vi "Roll station.vi"(0 "configuration file path":path caption="配置文件的路径", 1 "Roll station msic inf":T1) -> ()   [LabVIEW 2014]
uses:
  Ctl.xio/Roll station msic ctl.ctl
  SubVIS.xio/DataSocket/DataSocket_Tags.ctl
  Ctl.xio/part type.ctl
  SubVIS.xio/Creat Write List VI's/DefCtrl/Station.ctl
  <vilib>/Utility/file.llb/Read From Spreadsheet File (string).vi
  SubVIS.xio/Hopper car inf/Curing inf.vi
  SubVIS.xio/DataSocket/Write PLC Vars/Write Dbl Var in.vi
  SubVIS.xio/DataSocket/Write PLC Vars/Write Bool Var in.vi
panel:
  in  "SQL information":string
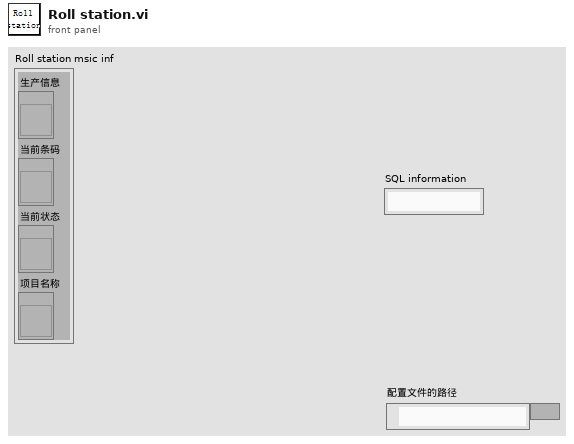
[diagram p1: front panel]
types:
  T1 = cluster{"生产信息":refnum<vi>, "当前条码":refnum<vi>, "当前状态":refnum<vi>, "项目名称":refnum<vi>}
  T2 = typedef "Station.ctl" = enum16{"粗切工位", "热处理工位", "精切工位", "PDF焊接工位", "打凹点预载力工位", "收卷工位", "EOL工位"}
  T3 = typedef "Roll station msic ctl.ctl" = cluster{"configuration file path":path, "DsOut":T4[], "Hopper car information":cluster{"Hopper car code":string, "Hopper car No":string, "plate No":string}, "pallet.produced number":i32, "SQL information":string, "Serial number":i32, "database path":path, "Roll station msic inf":cluster{"生产信息":refnum<vi>, "当前条码":refnum<vi>, "当前状态":refnum<vi>, "项目名称":refnum<vi>}, "part type":T5, "BarCode":string, "scanner resource name out":refnum<visa-resource-name>, "scanner coms or ip":string, "scanner ip ID":refnum<k5>, "curing timer":i32}
  T4 = typedef "DataSocket_Tags.ctl" = cluster{"Ds ID":refnum<k13>, "Tag":string}
  T5 = typedef "part type.ctl" = cluster{"项目号":string, "物料代码":string, "零件号":string, "供应商编码":string, "产线编码":string, "客户代码":string, "颜色代码":string, "托盘上限":i32, "加热温度":string, "加热时长":string, "EOL Stations":string}
  T6 = cluster{"Hopper car code":string, "Hopper car No":string, "plate No":string}
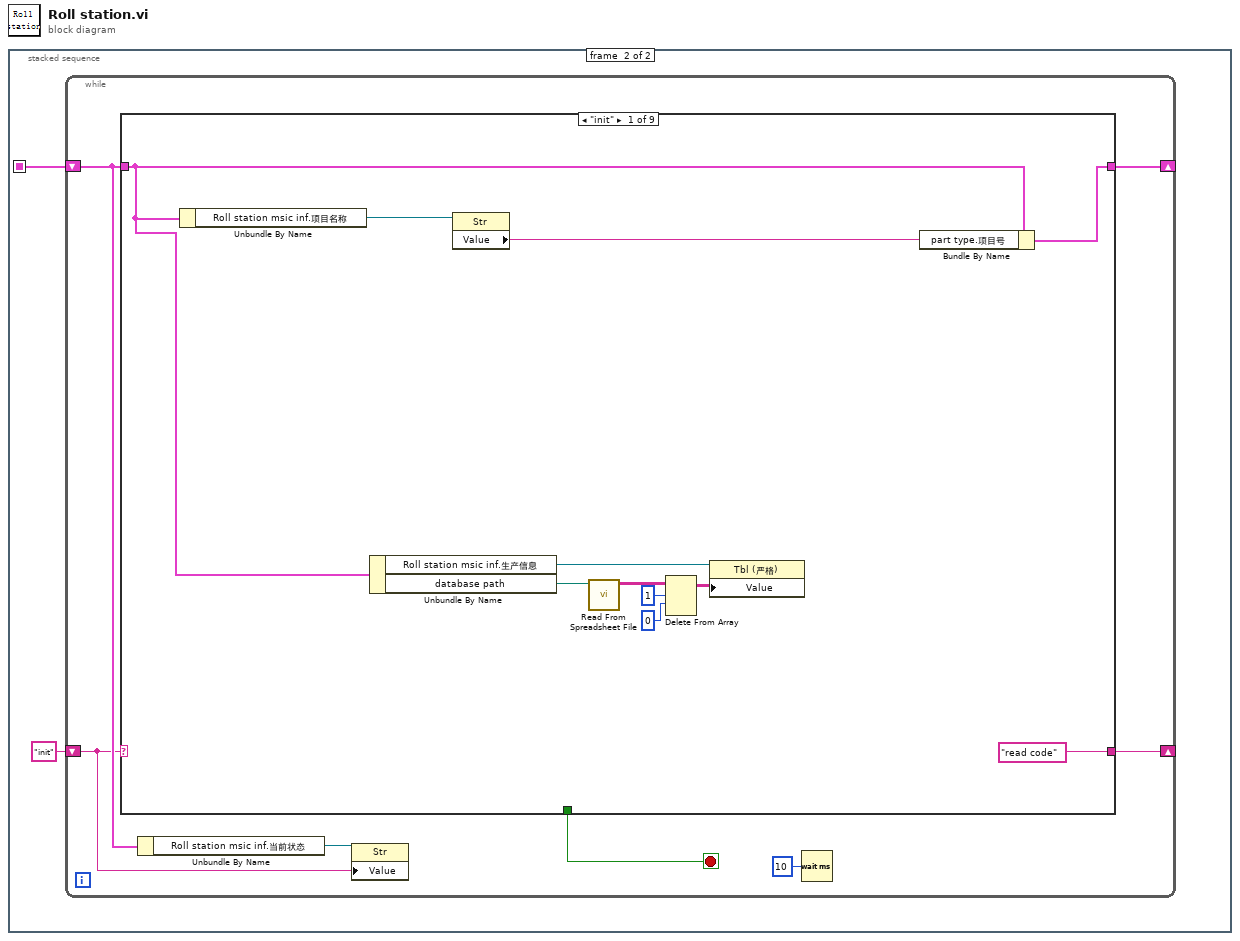
[diagram p0: block diagram]
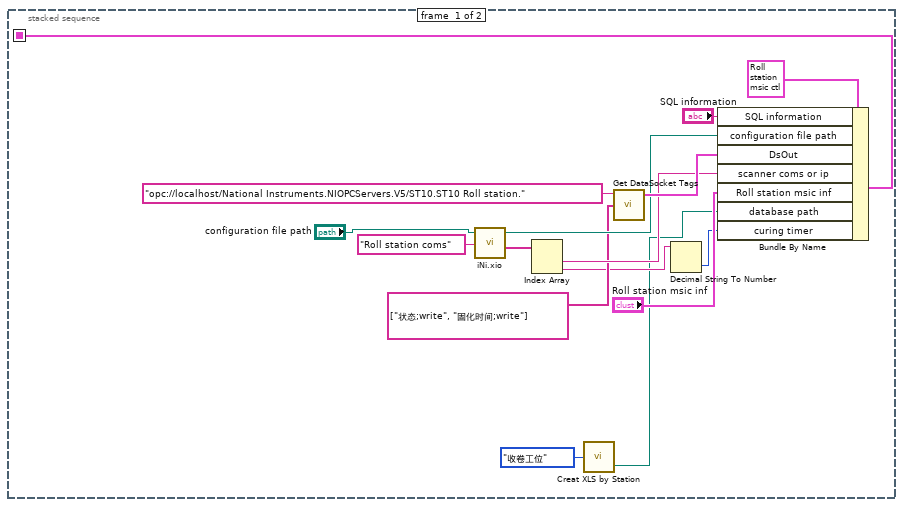
[diagram p2: hidden frame]
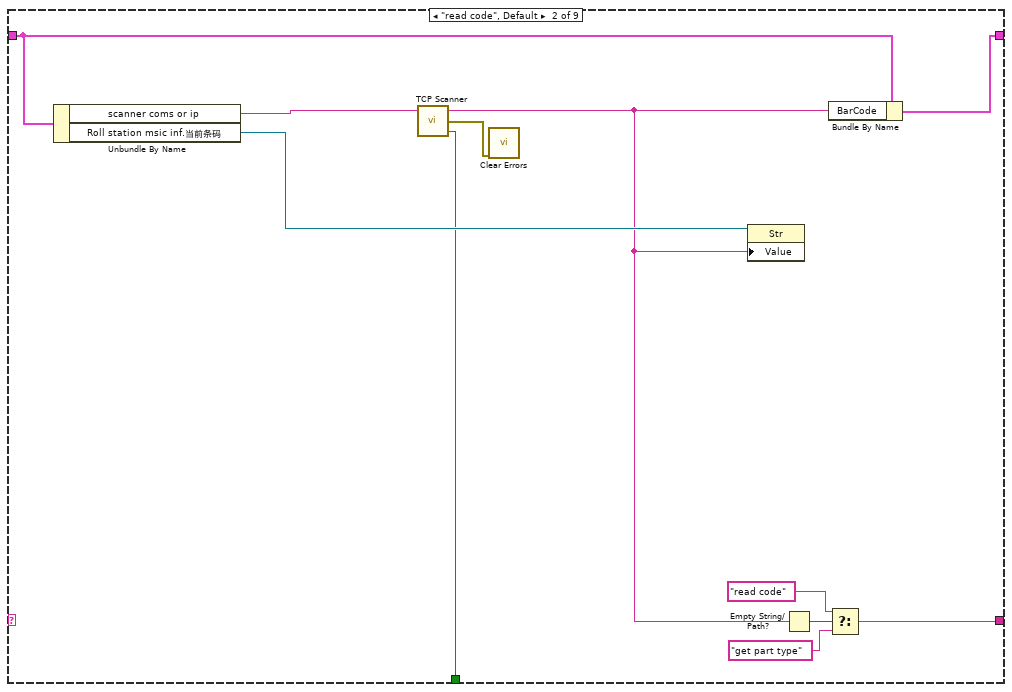
[diagram p3: hidden frame]
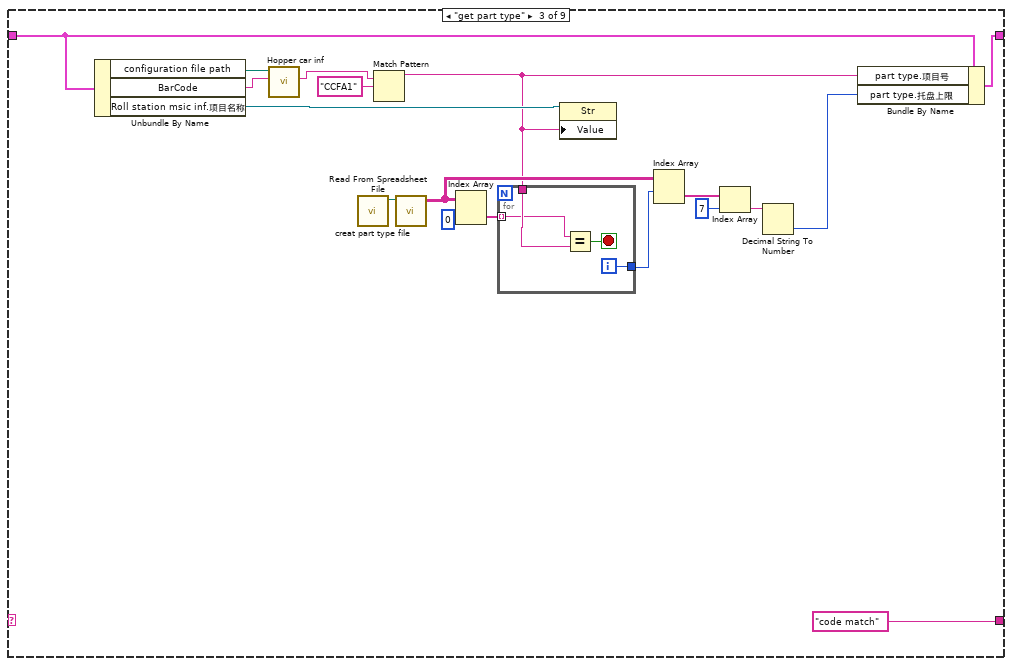
[diagram p4: hidden frame]
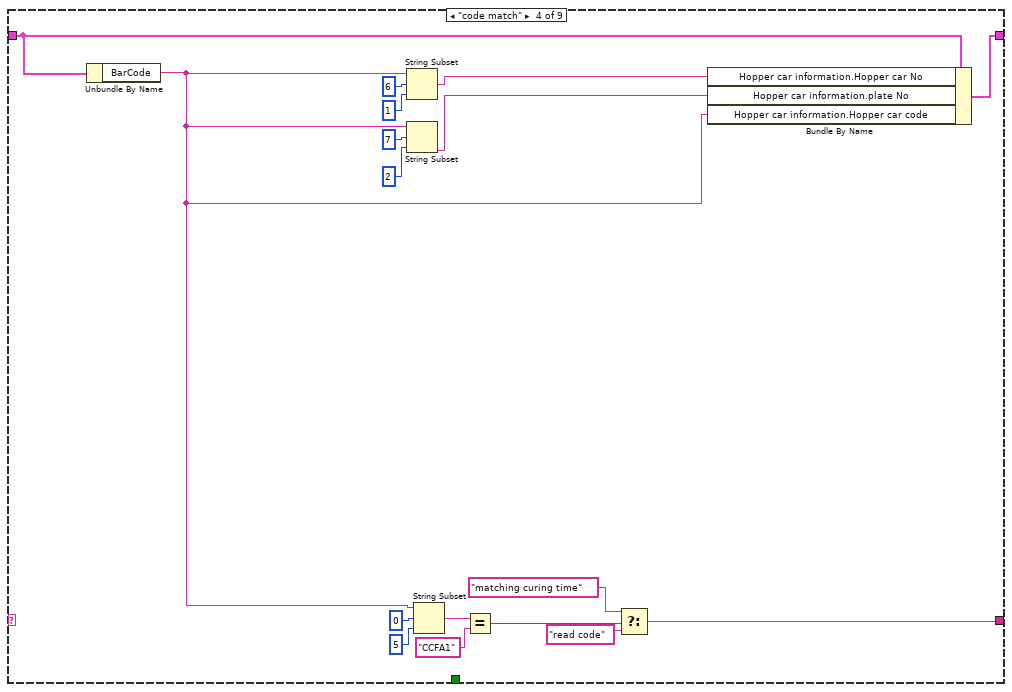
[diagram p5: hidden frame]
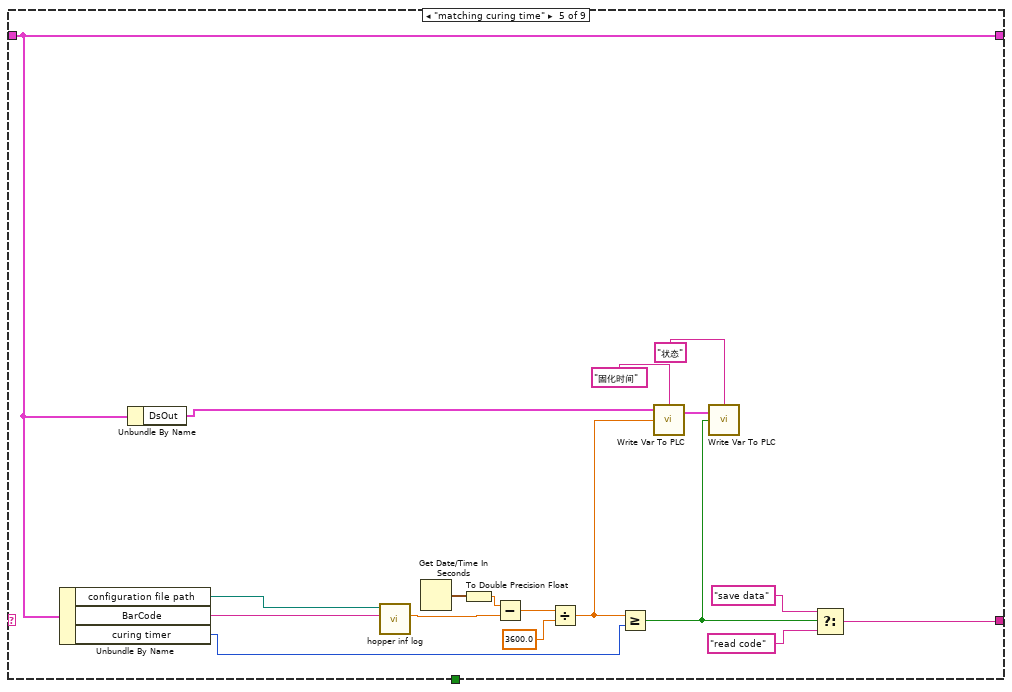
[diagram p6: hidden frame]
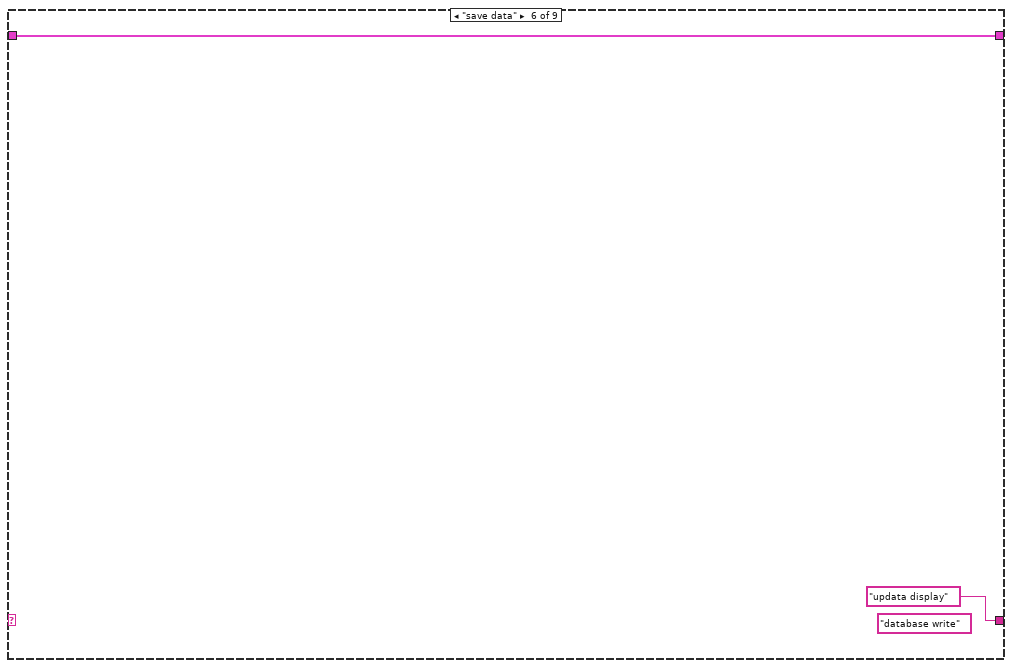
[diagram p7: hidden frame]
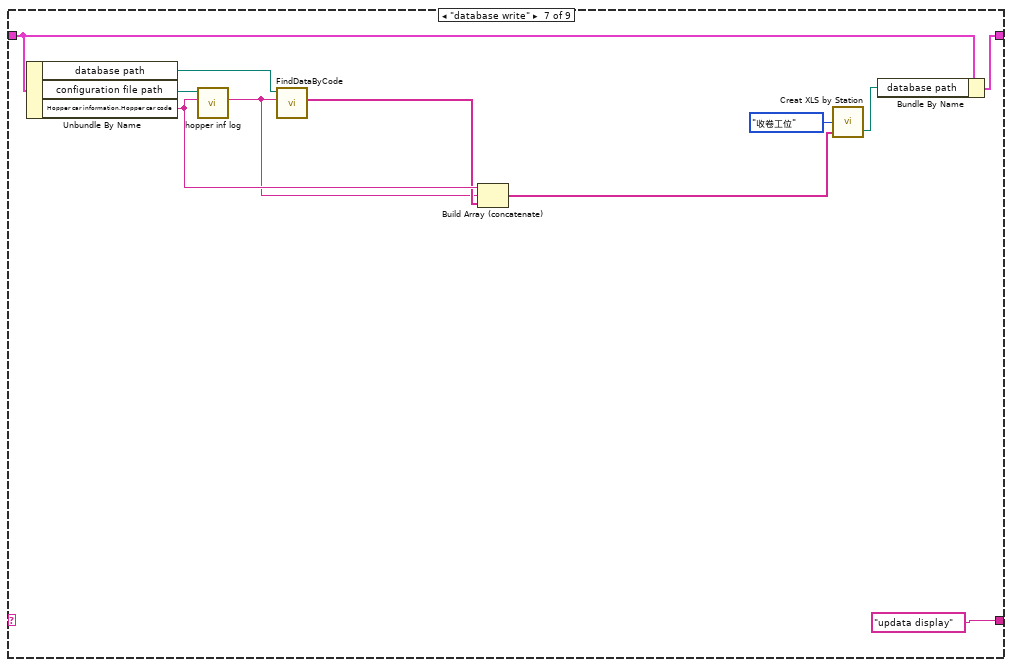
[diagram p8: hidden frame]
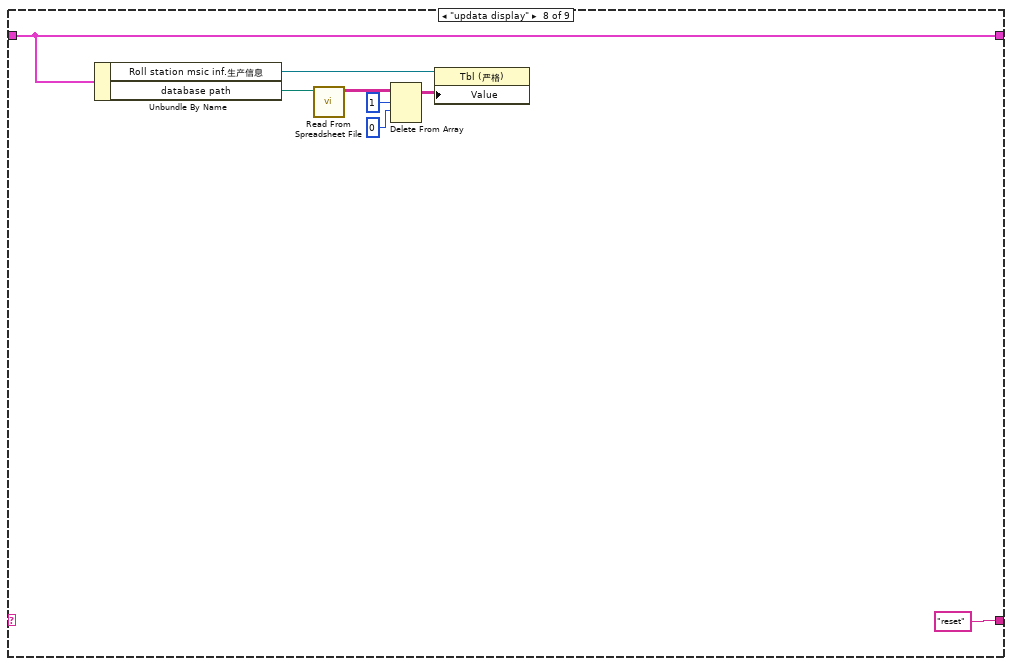
[diagram p9: hidden frame]
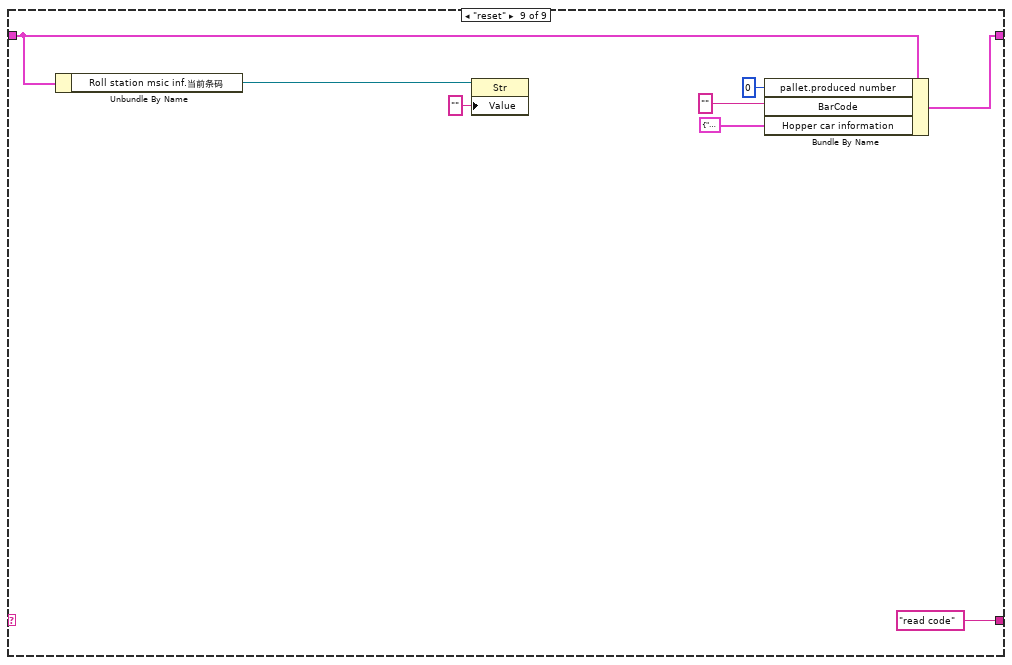
[diagram p10: hidden frame]
diagram:
  n1 = stacked-sequence {
    seq-local: [w7 _] -> [_ w18]
    frame #0 {
      n2 = call "iNi.xio.vi"("configuration file path"="configuration file path", "Sections"="Roll station coms") -> ("configuration file path"=w15:path, "Values"=w13:string[])  [unwired: 1 in, 3 out]
      n3 = Index Array(array=w13) -> (element #1=w12:string, element #2=w3:string)  [unwired: 2 in]
      n4 = call "Creat XLS by Station.vi"("staiton"=Station."收卷工位") -> ("new file path (Not A Path if cancelled)"=w2:path)  [unwired: 5 in]
      n5 = call "Get DataSocket Tags.vi"("All Tags"=string[] ["状态;write", "固化时间;write"], "URL"="opc://localhost/National Instruments.NIOPCServers.V5/ST10.ST10 Roll station.") -> ("DsOut"=w16:T4[])  [unwired: 3 in]
      n6 = Decimal String To Number(string=w3) -> (number=w4:i32)  [unwired: 2 in, 1 out]
      n7 = Bundle By Name(cluster=T3 {"configuration file path"=path "", "DsOut"=[], "Hopper car information"={"Hopper car code"="", "Hopper car No"="", "plate No"=""}, "pallet.produced number"=0, "SQL information"="", "Serial number"=0, "database path"=path "", "Roll station msic inf"={"生产信息"=refnum, "当前条码"=refnum, "当前状态"=refnum, "项目名称"=refnum}, "part type"={"项目号"="", "物料代码"="", "零件号"="", "供应商编码"="", "产线编码"="", "客户代码"="", "颜色代码"="", "托盘上限"=0, "加热温度"="", "加热时长"="", "EOL Stations"=""}, "BarCode"="", "scanner resource name out"="", "scanner coms or ip"="", "scanner ip ID"=refnum, "curing timer"=0} ("PDF Welding msic ctl"), "SQL information"="SQL information", "configuration file path"=w15, "DsOut"=w16, "scanner coms or ip"=w12, "Roll station msic inf"="Roll station msic inf", "database path"=w2, "curing timer"=w4) -> (w7:T3)
    }
    frame #1 {
      n8 = while {
        shift-right: [w25] -> _
        shift-left: w18 -> [w21]
        shift-right: [w24] -> _
        shift-left: "init" ("f") -> [w20]
        stop <- w19 stop-if-true
        n9 = case shown="\"init\"" w20 {
          tunnel: w21 -> [w26 w45 w51 w72 w93 w105 w115 w122 w128]
          tunnel: [w36 w47 w65 w80 w93 w105 w116 w122 w132] -> w25
          tunnel: ["read code" w39 "code match" w79 w98 "updata display" ("f") "updata display" ("f") "reset" ("f") "read code" ("f")] -> w24
          tunnel: [_ w37 _ _ _ _ _ _ _] -> w19
          frame "init" {
            n10 = Unbundle By Name(w26) -> ("Roll station msic inf.项目名称"=w35:refnum<vi>)
            n11 = Unbundle By Name(w26) -> ("Roll station msic inf.生产信息"=w32:refnum<vi>, "database path"=w31:path)
            n12 = property class="Str"(reference=w35) -> ("Value"=w34:string)  [unwired: 1 in, 2 out]
            n13 = call-poly <vilib>:"Read From Spreadsheet File.vi"("file path (dialog if empty)"=w31) -> ("all rows"=w30:string[][])  [unwired: 6 in, 4 out]
            n14 = Delete From Array(array=w30, length=1 ("长度"), index (row)=0 ("索引 (行)")) -> (array with subset deleted=w27:string[][])  [unwired: 1 in, 1 out]
            n15 = property class="Tbl (严格)"(reference=w32, "Value"=w27) -> ()  [unwired: 1 in, 2 out]
            n16 = Bundle By Name(cluster=w26, "part type.项目号"=w34) -> (w36:T3)
          }
          frame "read code", Default {
            n17 = Unbundle By Name(w45) -> ("scanner coms or ip"=w44:string, "Roll station msic inf.当前条码"=w46:refnum<vi>)
            n18 = call "TCP Scanner.vi"("ip"=w44) -> ("status"=w37:bool, "错误输出"=w43:errorcluster, "Barcode"=w38:string)  [unwired: 2 in]
            n19 = call <vilib>:"Clear Errors.vi"("error in (no error)"=w43) -> ()  [unwired: 5 in, 2 out]
            n20 = property class="Str"(reference=w46, "Value"=w38) -> ()  [unwired: 1 in, 2 out]
            n21 = Empty String/Path?(string/path=w38) -> (empty?=w42:bool)
            n22 = Bundle By Name(cluster=w45, "BarCode"=w38) -> (w47:T3)
            n23 = Select(t="read code", s=w42, f="get part type") -> (s? t:f=w39:string)
          }
          frame "get part type" {
            n24 = Unbundle By Name(w51) -> ("configuration file path"=w55:path, "BarCode"=w54:string, "Roll station msic inf.项目名称"=w50:refnum<vi>)
            n25 = call "Hopper car inf.vi"("key"=w54, "path in"=w55) -> ("value out"=w53:string)  [unwired: 8 in, 1 out]
            n26 = call "creat part type file.vi"() -> ("new file path (Not A Path if cancelled)"=w56:path)  [unwired: 11 in]
            n27 = Match Pattern(string=w53, regular expression="CCFA1" ("正则表达式")) -> (before substring=w49:string)  [unwired: 1 in, 3 out]
            n28 = call-poly <vilib>:"Read From Spreadsheet File.vi"("file path (dialog if empty)"=w56) -> ("all rows"=w61:string[][])  [unwired: 6 in, 4 out]
            n29 = Index Array(array=w61, index (col)=0 ("禁用的索引 (列)")) -> (element=w63:string[])  [unwired: 1 in]
            n30 = for {
              tunnel: w63 -> [w66] mode=indexing
              tunnel: [w68] -> w60
              tunnel: w49 -> [w67]
              i -> [w68]
              stop <- w69 stop-if-true
              n31 = Equal?(x=w66, y=w67) -> (x = y?=w69:bool)
            }
            n32 = property class="Str"(reference=w50, "Value"=w49) -> ()  [unwired: 1 in, 2 out]
            n33 = Index Array(array=w61, index (row)=w60) -> (element=w59:string[])  [unwired: 1 in]
            n34 = Index Array(array=w59, index=7 ("索引")) -> (element=w58:string)
            n35 = Decimal String To Number(string=w58) -> (number=w57:i32)  [unwired: 2 in, 1 out]
            n36 = Bundle By Name(cluster=w51, "part type.项目号"=w49, "part type.托盘上限"=w57) -> (w65:T3)
          }
          frame "code match" {
            n37 = Unbundle By Name(w72) -> ("BarCode"=w71:string)
            n38 = String Subset(string=w71, offset (0)=6 ("偏移量(0)"), length (rest)=1 ("长度（剩余）")) -> (substring=w74:string)
            n39 = String Subset(string=w71, offset (0)=7 ("偏移量(0)"), length (rest)=2 ("长度（剩余）")) -> (substring=w75:string)
            n40 = String Subset(string=w71, offset (0)=0 ("偏移量(0)"), length (rest)=5 ("长度（剩余）")) -> (substring=w76:string)
            n41 = Equal?(x=w76, y="CCFA1") -> (x = y?=w70:bool)
            n42 = Select(t="matching curing time" ("event"), s=w70, f="read code" ("event")) -> (s? t:f=w79:string)
            n43 = Bundle By Name(cluster=w72, "Hopper car information.Hopper car No"=w74, "Hopper car information.plate No"=w75, "Hopper car information.Hopper car code"=w71) -> (w80:T3)
          }
          frame "matching curing time" {
            n44 = Unbundle By Name(w93) -> ("configuration file path"=w104:path, "BarCode"=w103:string, "curing timer"=w96:i32)
            n45 = Unbundle By Name(w93) -> ("DsOut"=w92:T4[])
            n46 = call-poly "hopper inf log.vi"("key"=w103, "path in"=w104) -> ("value out"=w94:dbl)  [unwired: 8 in, 1 out]
            n47 = Get Date/Time In Seconds() -> (seconds since 1Jan1904=w102:timestamp)
            n48 = To Double Precision Float(number=w102) -> (double precision float=w95:dbl)
            n49 = Subtract(x=w95, y=w94) -> (x-y=w101:dbl)
            n50 = Divide(x=w101, y=3600.0) -> (x/y=w88:dbl)
            n51 = Greater Or Equal?(x=w88, y=w96) -> (x >= y?=w87:bool)
            n52 = call-poly "Write Var To PLC.vi"("Tag IN"="固化时间", "Dbl Var in"=w88, "Ds PLCTags IN"=w92) -> ("Ds PLCTags OUT"=w90:T4[])  [unwired: 1 in, 1 out]
            n53 = call-poly "Write Var To PLC.vi"("Tag IN"="状态", "Bool Var in"=w87, "Ds PLCTags IN"=w90) -> ()  [unwired: 1 in, 2 out]
            n54 = Select(t="save data" ("event"), s=w87, f="read code") -> (s? t:f=w98:string)
          }
          frame "save data" {
            (unwired) "database write" ("f")
          }
          frame "database write" {
            n55 = Unbundle By Name(w115) -> ("database path"=w111:path, "configuration file path"=w114:path, "Hopper car information.Hopper car code"=w110:string)
            n56 = call-poly "hopper inf log.vi"("key"=w110, "path in"=w114) -> ("value out"=w107:string)  [unwired: 8 in, 1 out]
            n57 = call "FindDataByCode.vi"("Code"=w107, "Database Path"=w111) -> ("all rows"=w108:string[])  [unwired: 9 in]
            n58 = Build Array (concatenate)(w110, w107, w108) -> (w109:string[])
            n59 = call "Creat XLS by Station.vi"("staiton"=Station."收卷工位", "data in"=w109) -> ("new file path (Not A Path if cancelled)"=w113:path)  [unwired: 4 in]
            n60 = Bundle By Name(cluster=w115, "database path"=w113) -> (w116:T3)
          }
          frame "updata display" {
            n61 = Unbundle By Name(w122) -> ("Roll station msic inf.生产信息"=w124:refnum<vi>, "database path"=w123:path)
            n62 = call-poly <vilib>:"Read From Spreadsheet File.vi"("file path (dialog if empty)"=w123) -> ("all rows"=w121:string[][])  [unwired: 6 in, 4 out]
            n63 = Delete From Array(array=w121, length=1 ("长度"), index (row)=0 ("索引 (行)")) -> (array with subset deleted=w118:string[][])  [unwired: 1 in, 1 out]
            n64 = property class="Tbl (严格)"(reference=w124, "Value"=w118) -> ()  [unwired: 1 in, 2 out]
          }
          frame "reset" {
            n65 = Unbundle By Name(w128) -> ("Roll station msic inf.当前条码"=w127:refnum<vi>)
            n66 = property class="Str"(reference=w127, "Value"="" ("值")) -> ()  [unwired: 1 in, 2 out]
            n67 = Bundle By Name(cluster=w128, "pallet.produced number"=0, "BarCode"="", "Hopper car information"=T6 {"Hopper car code"="", "Hopper car No"="", "plate No"=""}) -> (w132:T3)
          }
        }
        n68 = Unbundle By Name(w21) -> ("Roll station msic inf.当前状态"=w22:refnum<vi>)
        n69 = property class="Str"(reference=w22, "Value"=w20) -> ()  [unwired: 1 in, 2 out]
        n70 = Wait (ms)(milliseconds to wait=u32 10 ("等待时间（毫秒）")) -> ()  [unwired: 1 out]
      }
    }
  }
